vi "Read Initialized.vi"(8 "error in (no error)":errorcluster, 11 "MB Data Block in":refnum<class "MB Data Block.lvclass">) -> (0 "error out":errorcluster, 2 "Initialized":bool, 3 "MB Data Block out":refnum<class "MB Data Block.lvclass">)   [LabVIEW 2018, in "MB PLC Client.lvlib" / "MB Data Block.lvclass"]
uses:
  MB Data Block.lvclass
  MB Data Block.lvclass/MB Data Block.ctl
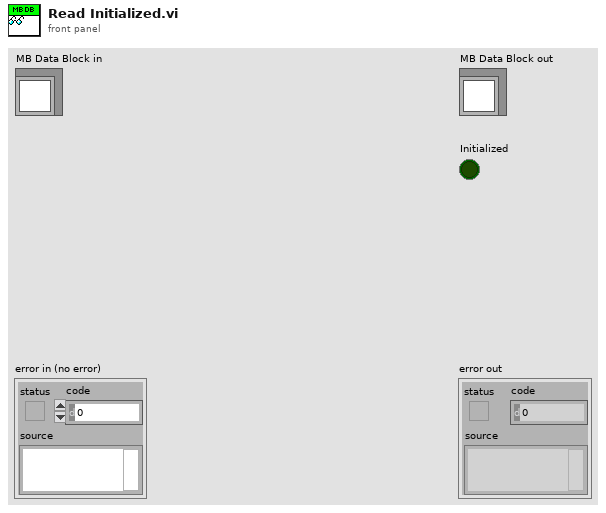
[diagram p1: front panel]
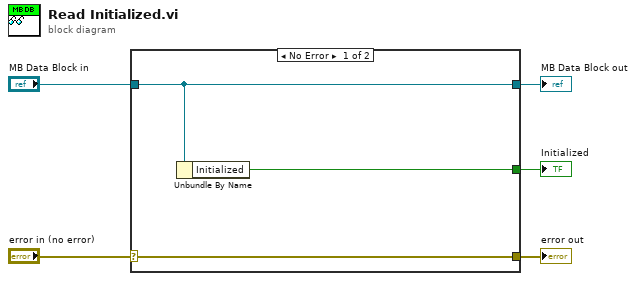
[diagram p0: block diagram]
diagram:
  n1 = case shown="No Error" "error in (no error)" {
    selector: "error in (no error)" -> [w8 w9]
    tunnel: [w8 w9] -> w4
    tunnel: [w7 w10] -> w2
    tunnel: "MB Data Block in" -> [w7 w10]
    tunnel: [w6 _] -> w1
    frame No Error {
      n2 = Unbundle By Name(w7) -> ("Initialized"=w6:bool)
    }
    frame Error {
    }
  }
  "error out" <- w4
  "MB Data Block out" <- w2
  "Initialized" <- w1
